vi "CommaToDot.vi"(1 "Input":T1) -> (0 "Output":T1)   [LabVIEW 2011]
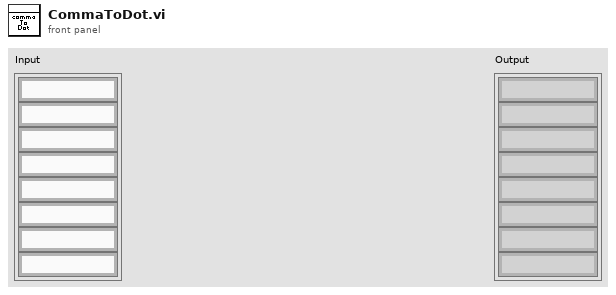
[diagram p1: front panel]
types:
  T1 = cluster{string, string, string, string, string, string, string, string}
  T2 = cluster{string, string, string, string, "result string":string, string, string, string}
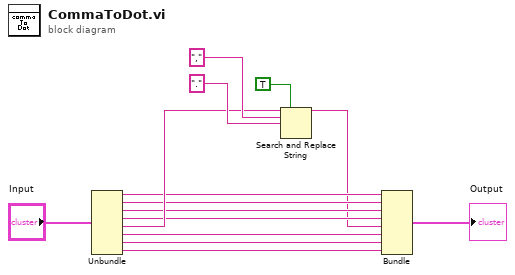
[diagram p0: block diagram]
diagram:
  n1 = Unbundle("Input") -> (w9:string, w8:string, w7:string, w6:string, w10:string, w5:string, w4:string, w3:string)
  n2 = Search and Replace String(replace all?=TRUE ("replace all? (F)"), input string=w10, search string=",", replace string="." ("replace string (\"\")")) -> (result string=w2:string)  [unwired: 4 in, 3 out]
  n3 = Bundle(w9, w8, w7, w6, "result string"=w2, w5, w4, w3) -> (→"Output":T2)  [unwired: 1 in]
